vi "QueryStatus.vi"(8 "Error In":errorcluster, 11 "Thorlabs In":refnum<class "Thorlabs.lvclass">) -> (0 "Error Out":errorcluster, 3 "Thorlabs Out":refnum<class "Thorlabs.lvclass">)   [LabVIEW 2018, in "Thorlabs.lvlib" / "Thorlabs.lvclass"]
doc: "This VI Queries the Status of the Axis Controller. \n\nCreator: Slade Jeppesen\nCreated Date: 09/29/20"
uses:
  Thorlabs.lvclass
  Thorlabs.lvclass/Thorlabs.ctl
  C:/AME Test Engineering/LabVIEW/PPLs/Axis/DLLs/ThorLabs.MotionControl.KCube.DCServoCLI.dll
  PPLs/Axis/DLLs/ThorLabs.MotionControl.KCube.DCServoCLI.dll
  C:/AME Test Engineering/LabVIEW/PPLs/Axis/DLLs/Thorlabs.MotionControl.GenericMotorCLI.dll
  PPLs/Axis/DLLs/Thorlabs.MotionControl.GenericMotorCLI.dll
  84b42895-8bc4-42c3-9f2d-1046c126a870.vi
  PPLs/Axis/Parent/Axis.lvlibp/Axis.lvclass
  C:/AME Test Engineering/LabVIEW/PPLs/Axis/Parent/Axis.lvlibp/Axis.lvclass
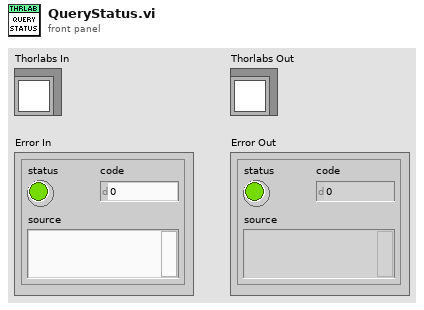
[diagram p1: front panel]
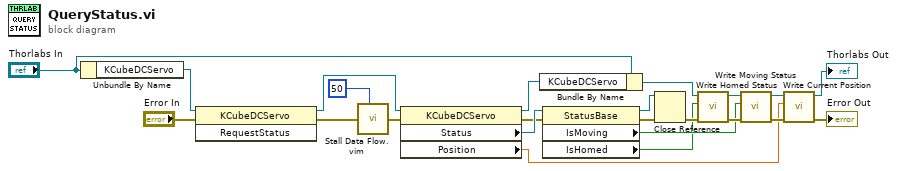
[diagram p0: block diagram]
diagram:
  n1 = Unbundle By Name("Thorlabs In") -> ("KCubeDCServo"=w23:refnum<k24>)
  n2 = invoke class="KCubeDCServo" method="RequestStatus"(reference=w23, error in="Error In") -> (reference out=w4:refnum<k24>, error out=w3:errorcluster)  [unwired: 1 in, 1 out]
  n3 = call "Stall Data Flow.vim"("value in"=w3, "milliseconds to wait"=u32 50) -> ("value out"=w17:errorcluster)  [unwired: 1 out]
  n4 = property class="KCubeDCServo"(reference=w4, error in=w17) -> (reference out=w15:refnum<k24>, error out=w18:errorcluster, "Status"=w21:refnum<k24>, "Position"=w2:dbl)
  n5 = Bundle By Name(cluster="Thorlabs In", "KCubeDCServo"=w15) -> (w7:refnum<class "Thorlabs.lvclass">)
  n6 = property class="StatusBase"(reference=w21, error in=w18) -> (reference out=w19:refnum<k24>, error out=w20:errorcluster, "IsMoving"=w5:bool, "IsHomed"=w1:bool)
  n7 = Close Reference(reference=w19, error in (no error)=w20) -> (error out=w6:errorcluster)
  n8 = call "Write Homed Status.vi"("error in (no error)"=w6, "Homed?"=w1, "Axis in"=w7) -> ("error out"=w9:errorcluster, "Axis out"=w11:refnum<class "Thorlabs.lvclass">)  [unwired: 7 in]
  n9 = call "Write Moving Status.vi"("error in (no error)"=w9, "Moving?"=w5, "Axis in"=w11) -> ("error out"=w8:errorcluster, "Axis out"=w10:refnum<class "Thorlabs.lvclass">)  [unwired: 7 in]
  n10 = call "Write Current Position.vi"("error in"=w8, "Current Position"=w2, "Axis in"=w10) -> ("error out"=→"Error Out":errorcluster, "Axis out"=→"Thorlabs Out":refnum<class "Thorlabs.lvclass">)  [unwired: 7 in]
